vi "Parameter.vi"(9 "In":string, 10 "VIId":string, 11 "VariablesRef":T1) -> ()   [LabVIEW 2018, in "Time.lvlib"]
uses:
  Time.lvlib
  <userlib>/_OpenG.lib/dictionary/dictionary.llb/Dictionary Object RefNum__ogtk.ctl
  <userlib>/_OpenG.lib/dictionary/dictionary.llb/Dictionary Object RefNum - Enum__ogtk.ctl
  <vilib>/addons/_JKI.lib/Serialization/JSON/JKI JSON Serialization.lvlib
panel:
  in  "Tab Control":enum32{"Config", "控件"}(tab)
  in  "ArrayType":enum32{"Wait_ms", "Wait_s", "TickCount"}(tab)
  in  "时间(ms)":i32
  in  "时间(s)":i32
  in  "方法(Method)":enum16{"Wait_ms", "Wait_s", "TickCount"}(ring)
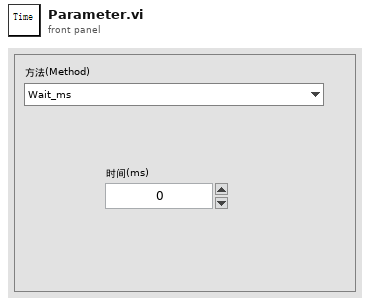
[diagram p1: front panel]
types:
  T1 = typedef "Dictionary Object RefNum__ogtk.ctl" = refnum<k1>
  T2 = cluster{"Wait_ms":cluster{"json":cluster{"Method":string, "Time":i32}}, "Wait_s":cluster{"json":cluster{"Method":string, "Time":i32}}, "TickCount":cluster{"json":cluster{"Method":string}}}
  T3 = enum32{"Invalid", "Standard", "Closed", "Hidden", "Minimized", "Maximized"}
  T4 = enum32{"invalid app kind", "Development System", "Run Time System", "Student Edition", "Embedded LabVIEW", "Evaluation", "Custom"}
  T5 = cluster{"Core":cluster{"Current VI Reference":refnum<vi>, "Close Panel on Exit?":bool}, "Parameter":cluster{"VariableRef":T1}, "Synchronize":cluster{"EnqueueData":cluster{"Action":enum16{"Create", "Query", "Revert", "UpdateVariable", "Close"}, "Data":variant}, "Echo":cluster{"VIRef":refnum<vi>, "JsonOut":string, "Status":string}, "Communicate":cluster{"ID":string, "JsonIn":string, "VarRef":T1}, "Queue":refnum<queue>}, "TimeClusters":cluster{"Wait_ms":cluster{"json":cluster{"Method":string, "Time":i32}}, "Wait_s":cluster{"json":cluster{"Method":string, "Time":i32}}, "TickCount":cluster{"json":cluster{"Method":string}}}}
  T6 = cluster{"EnqueueData":cluster{"Action":enum16{"Create", "Query", "Revert", "UpdateVariable", "Close"}, "Data":variant}, "Echo":cluster{"VIRef":refnum<vi>, "JsonOut":string, "Status":string}, "Communicate":cluster{"ID":string, "JsonIn":string, "VarRef":T1}, "Queue":refnum<queue>}
  T7 = cluster{"Current VI Reference":refnum<vi>, "Close Panel on Exit?":bool}
  T8 = cluster{"json":cluster{"Method":string, "Time":i32}}
  T9 = cluster{"Action":enum16{"Create", "Query", "Revert", "UpdateVariable", "Close"}, "Data":variant}
  T10 = cluster{"ID":string, "JsonIn":string, "VarRef":T1}
  T11 = enum16{"Create", "Query", "Revert", "UpdateVariable", "Close"}
  T12 = cluster{"VIRef":refnum<vi>, "JsonOut":string, "Status":string}
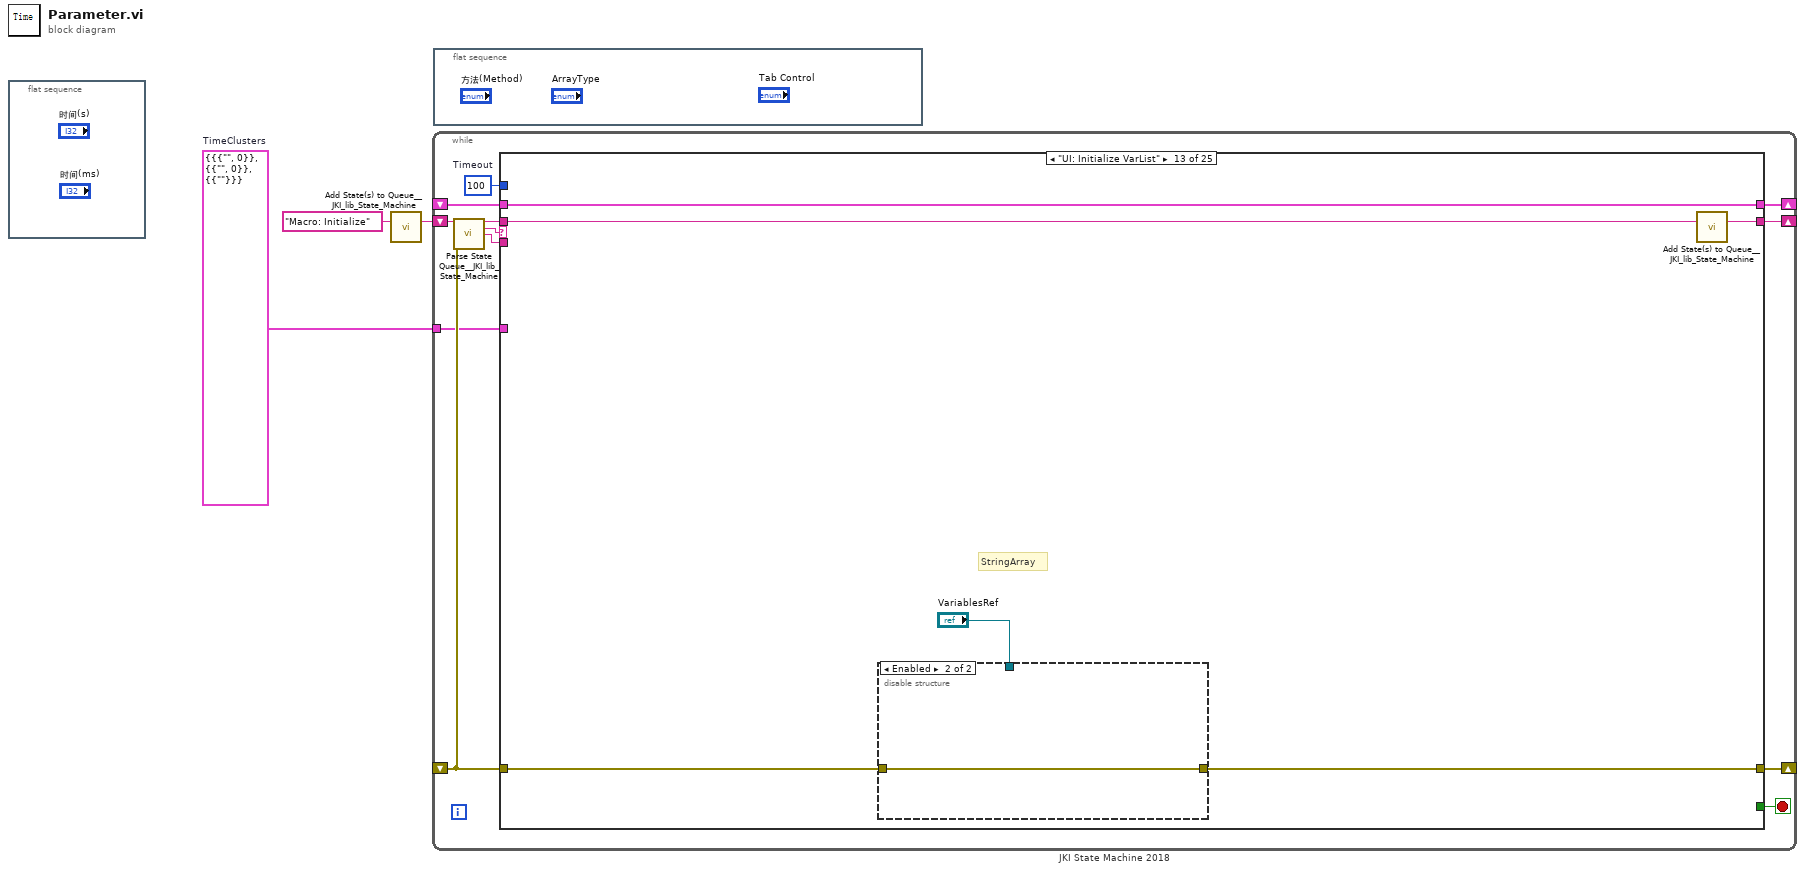
[diagram p0: block diagram]
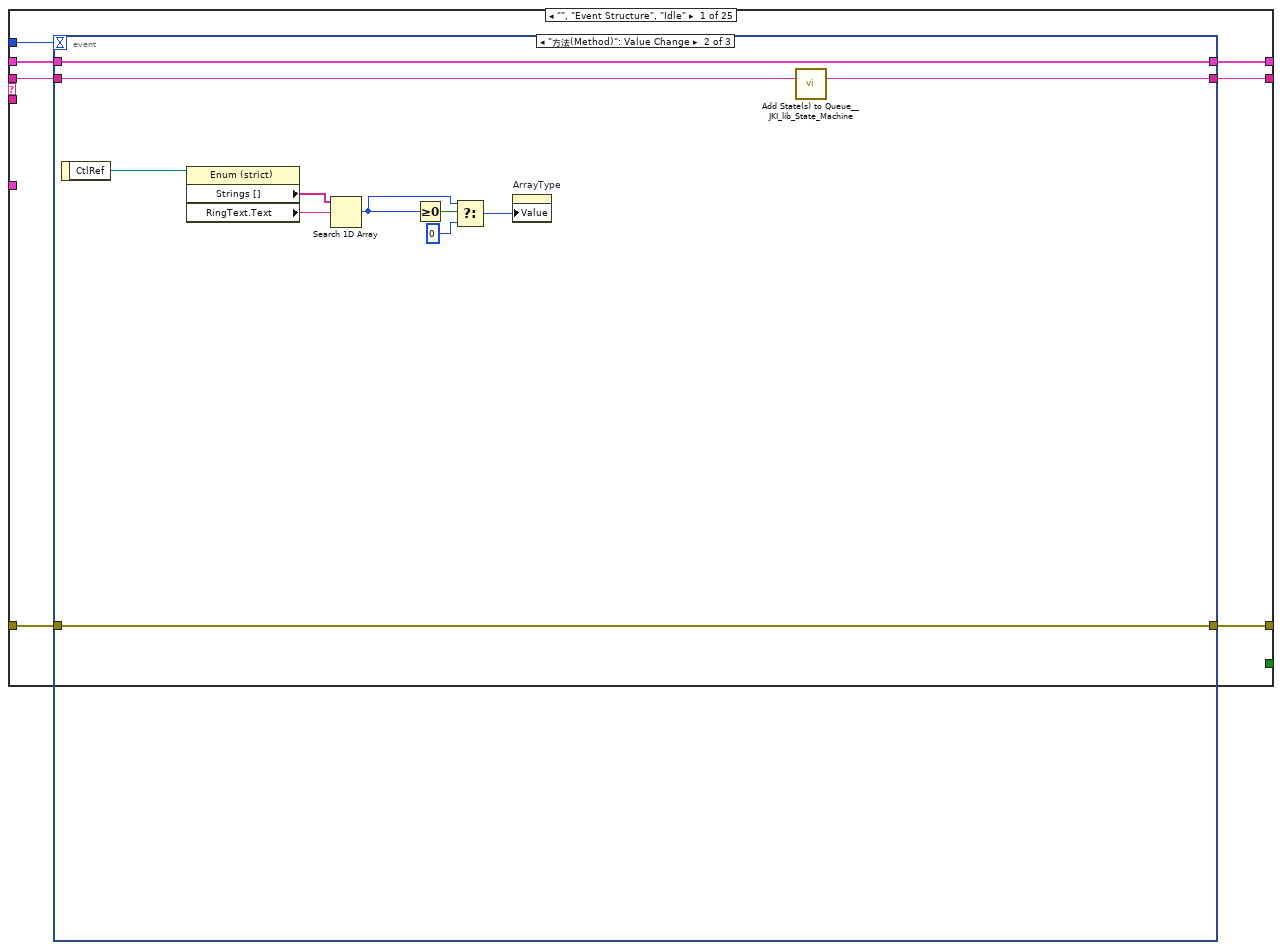
[diagram p2: hidden frame]
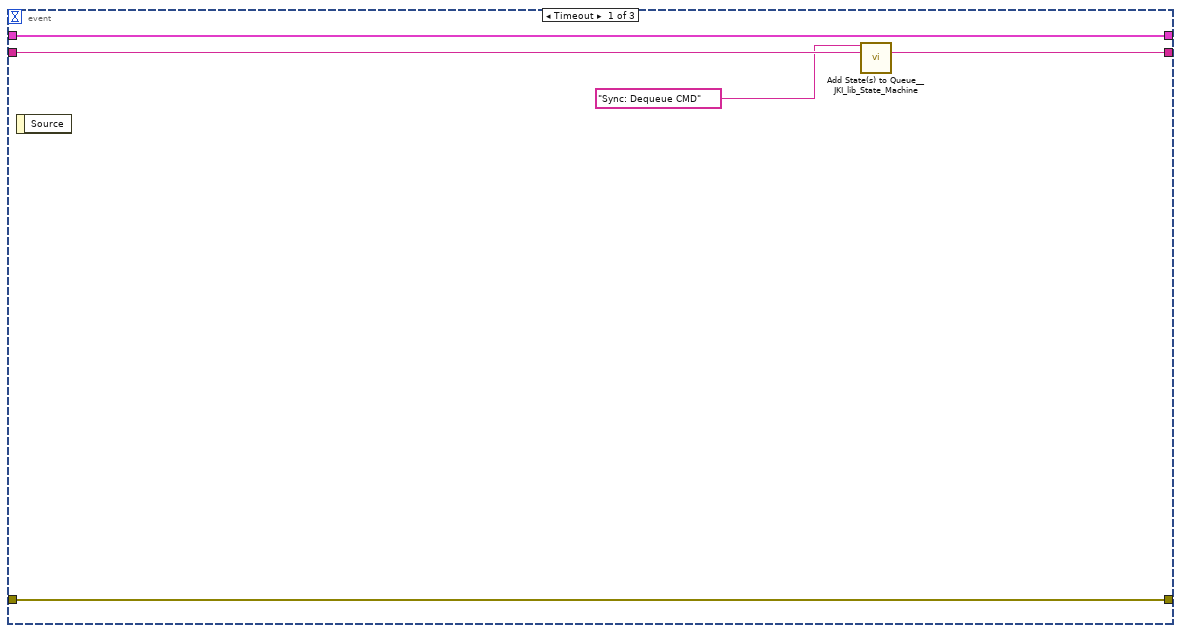
[diagram p3: hidden frame]
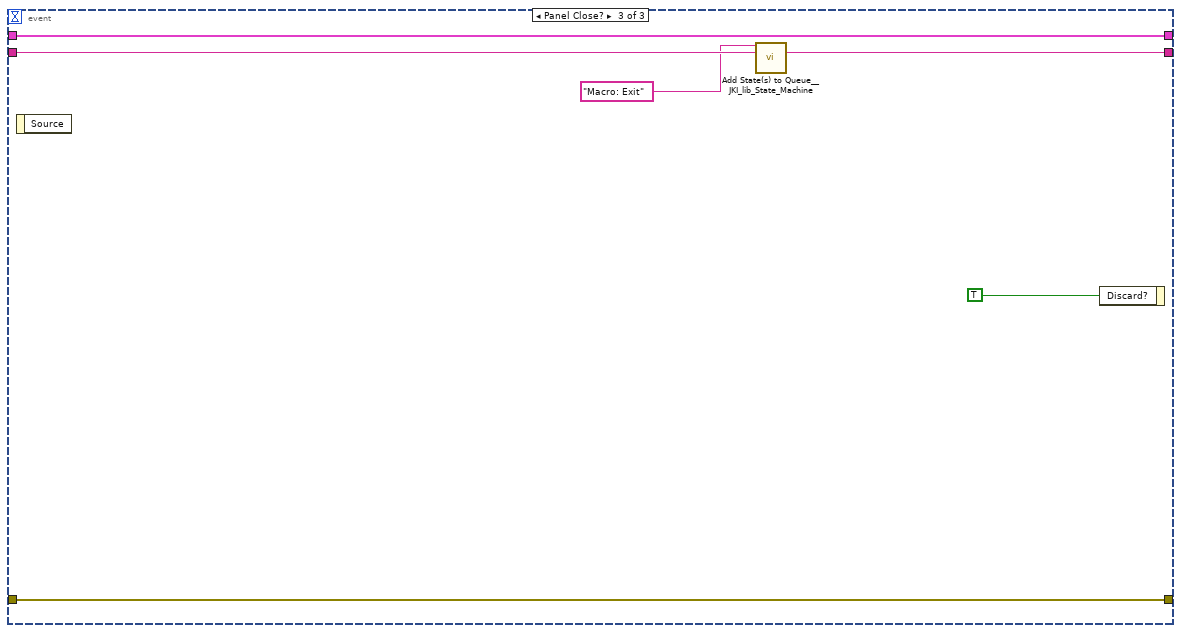
[diagram p4: hidden frame]
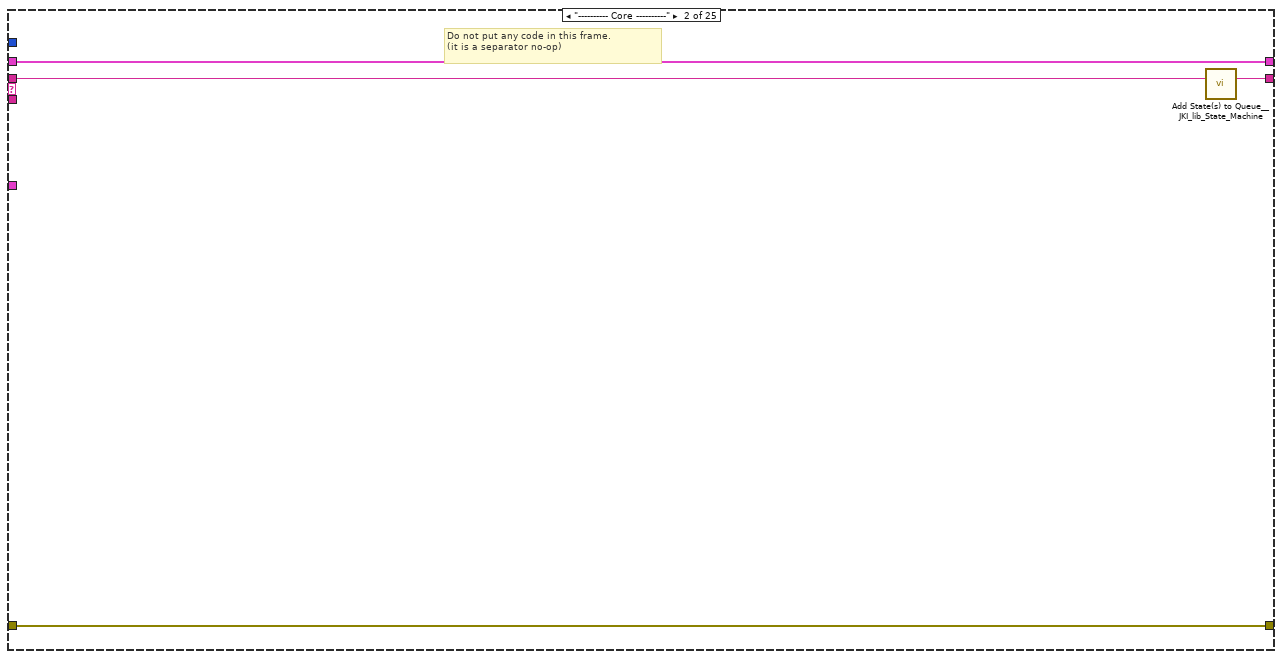
[diagram p5: hidden frame]
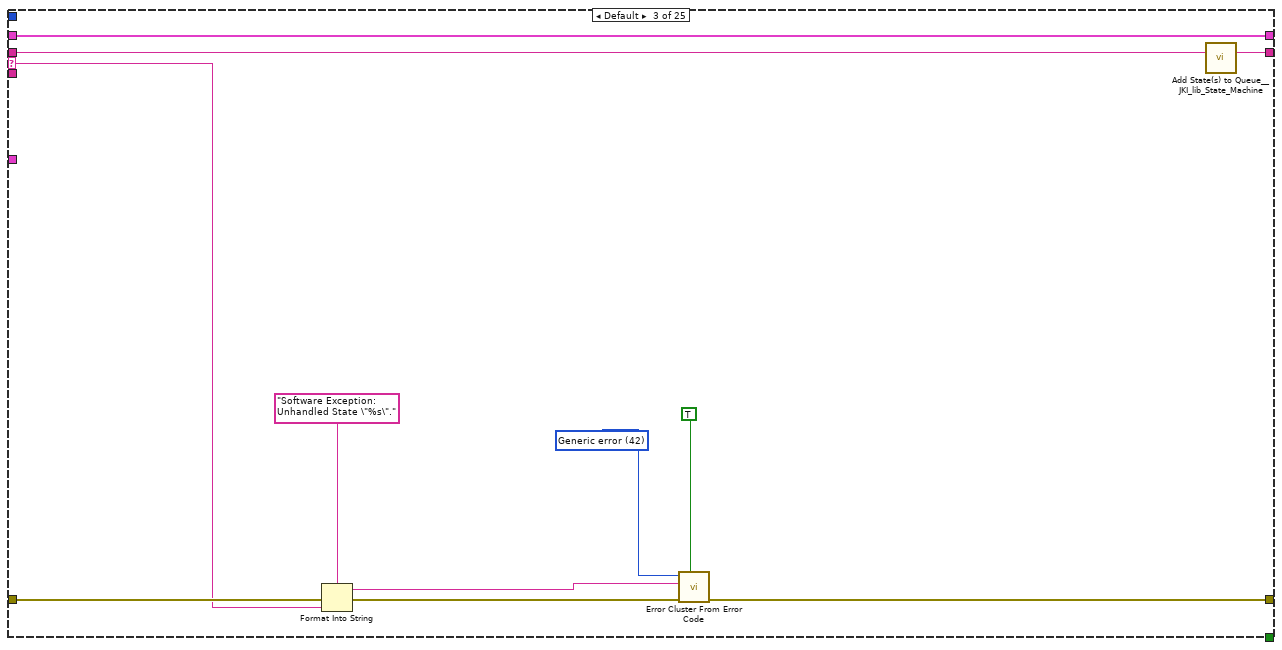
[diagram p6: hidden frame]
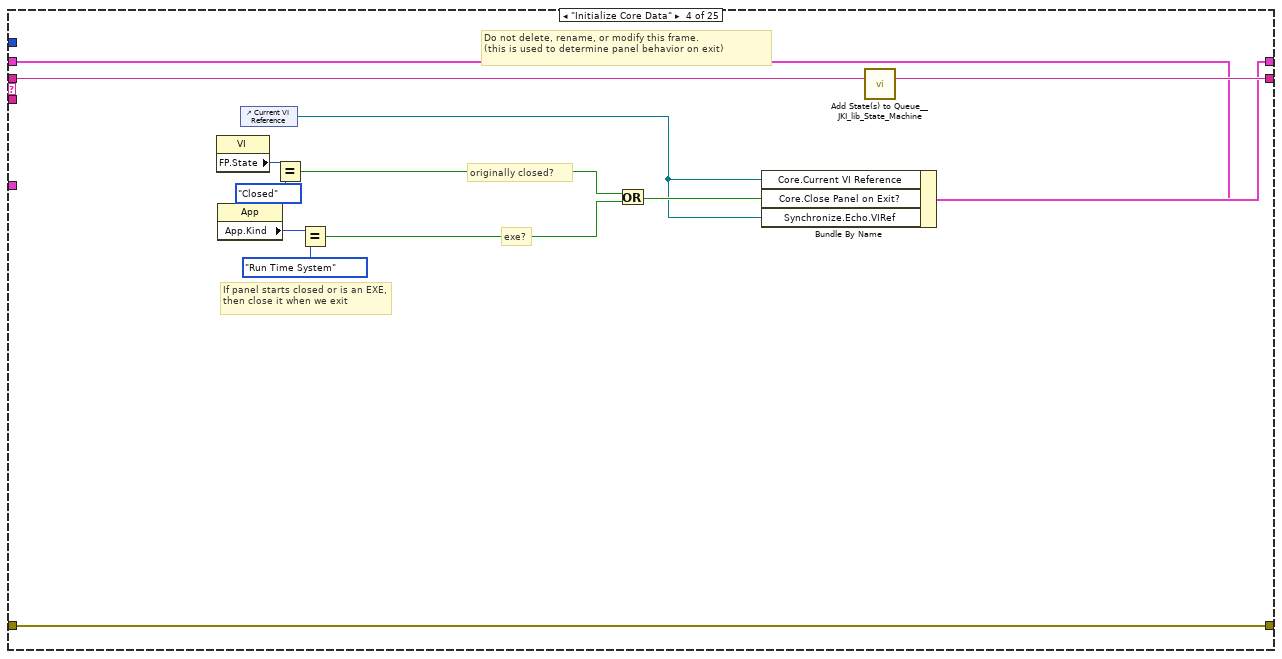
[diagram p7: hidden frame]
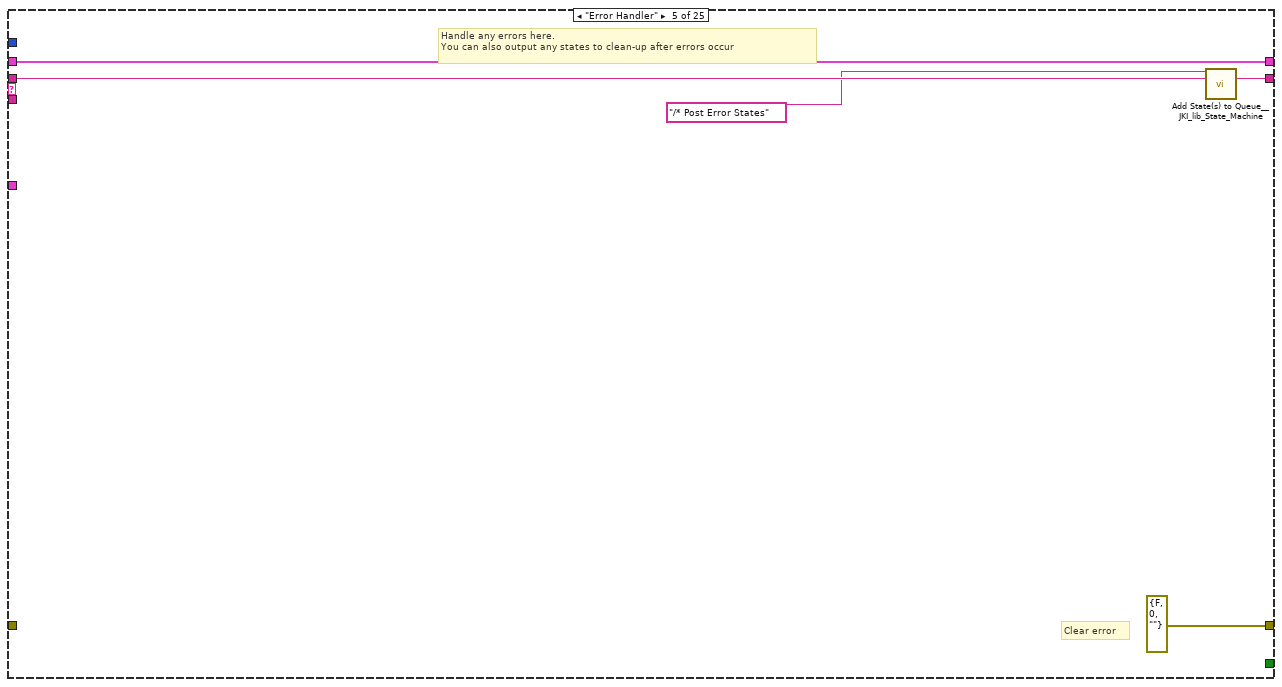
[diagram p8: hidden frame]
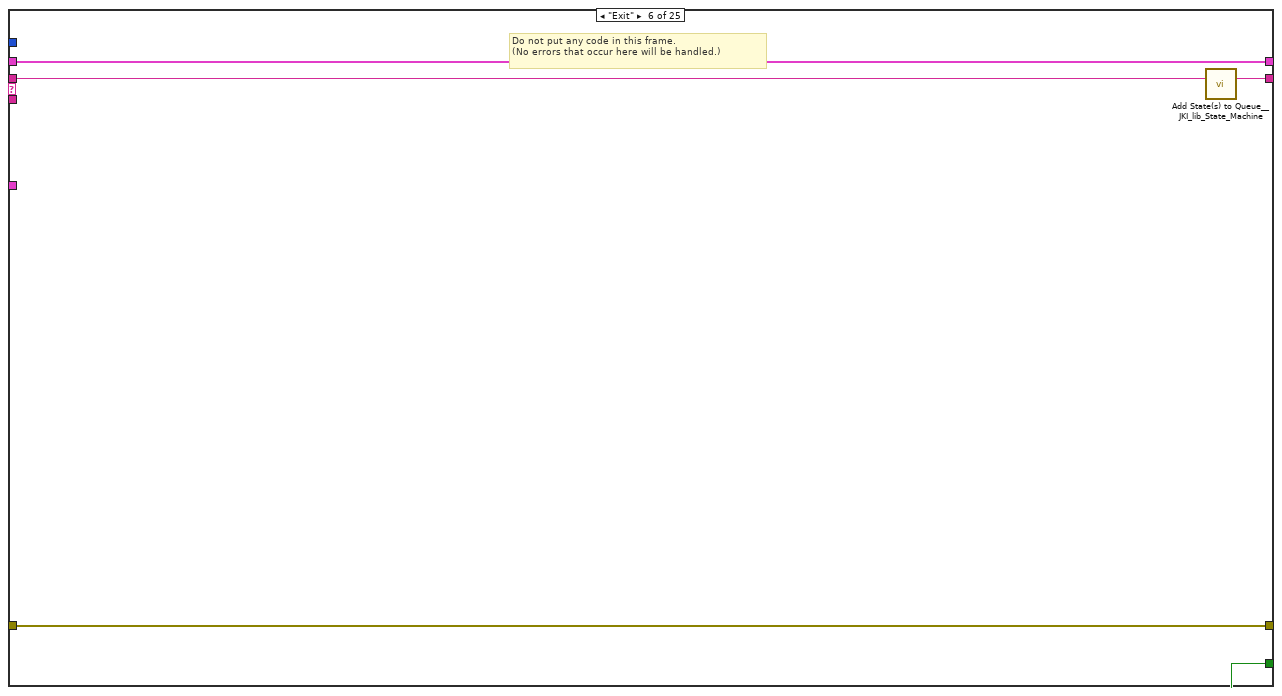
[diagram p9: hidden frame]
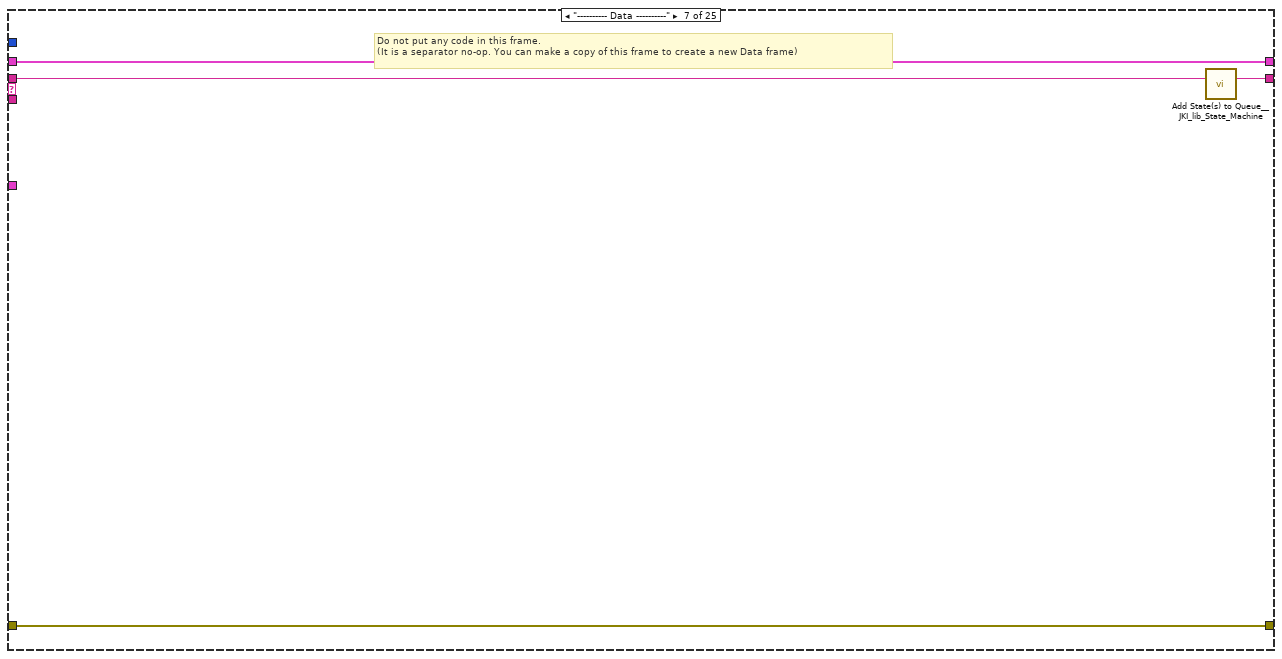
[diagram p10: hidden frame]
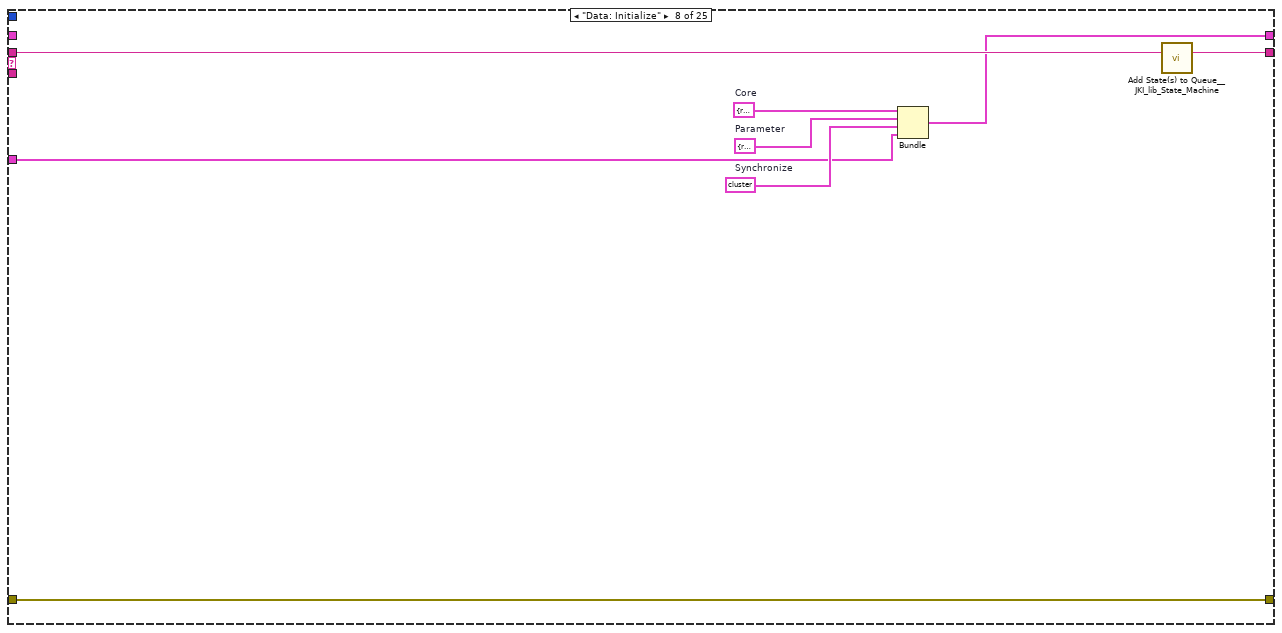
[diagram p11: hidden frame]
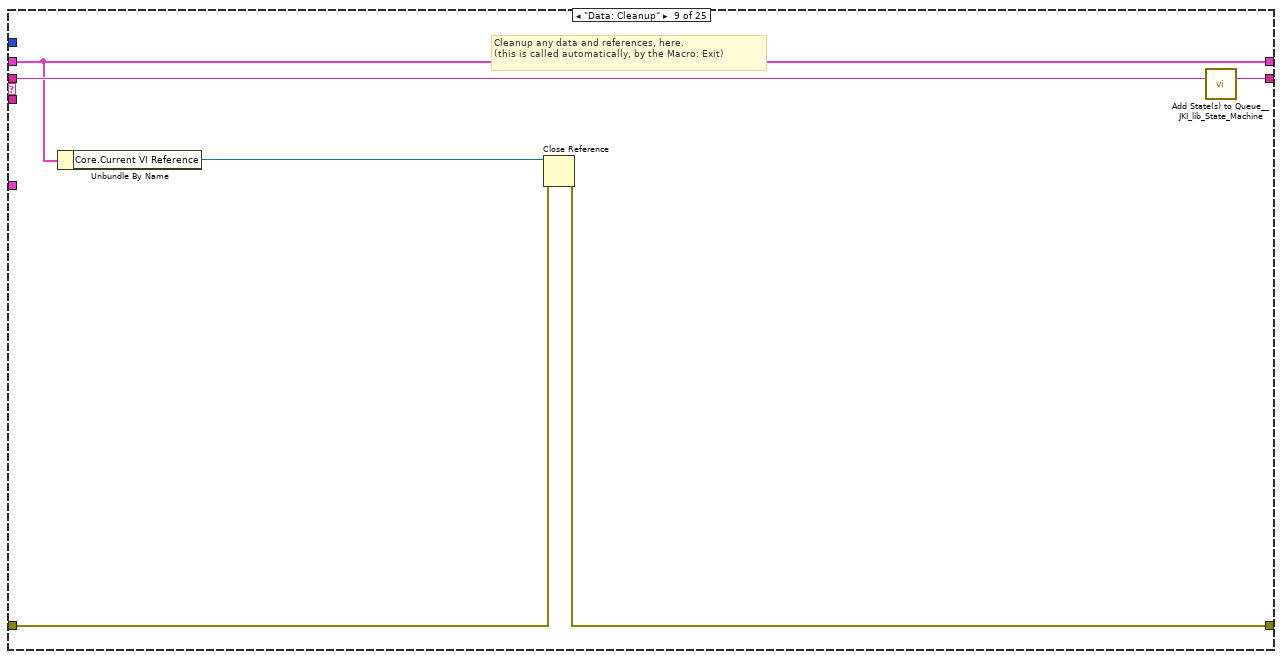
[diagram p12: hidden frame]
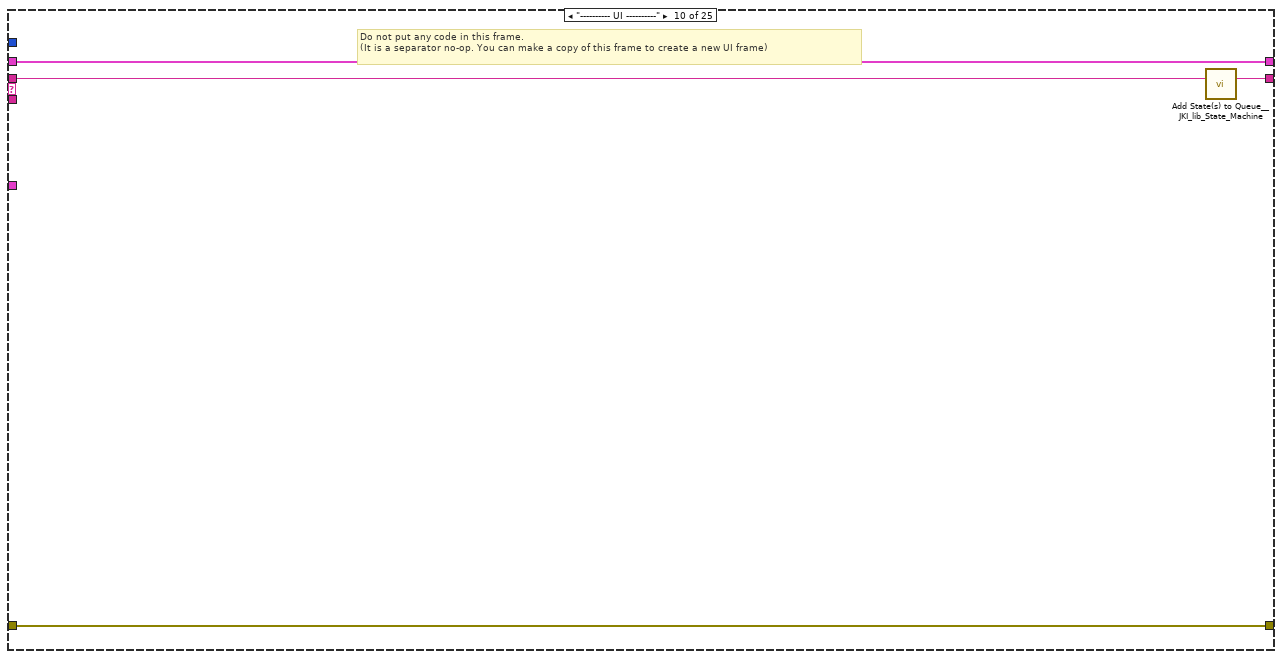
[diagram p13: hidden frame]
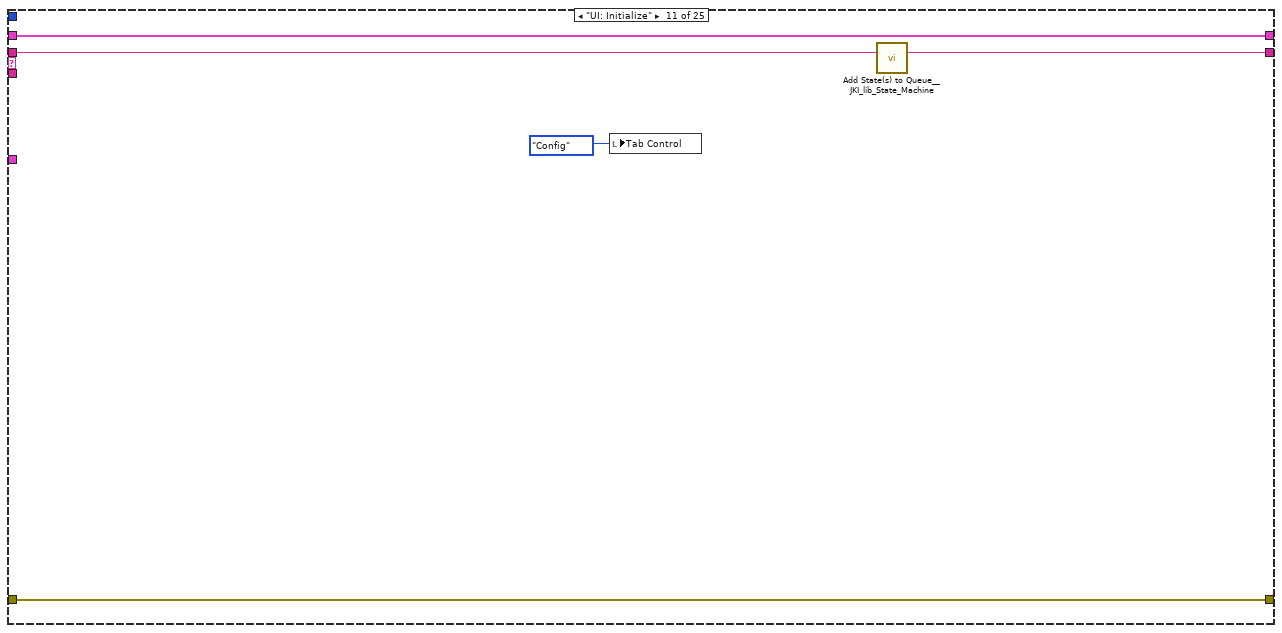
[diagram p14: hidden frame]
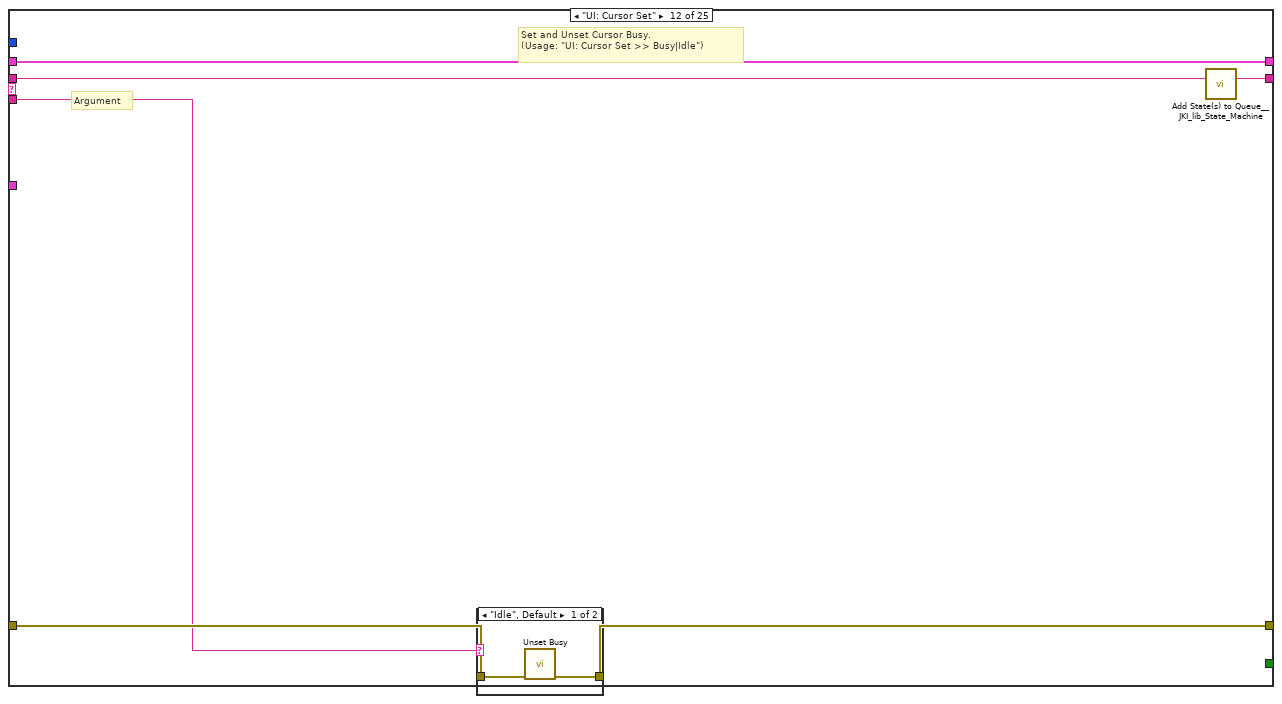
[diagram p15: hidden frame]
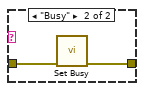
[diagram p16: hidden frame]
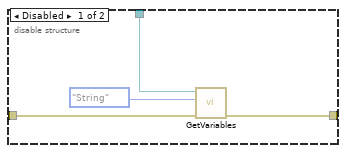
[diagram p17: hidden frame]
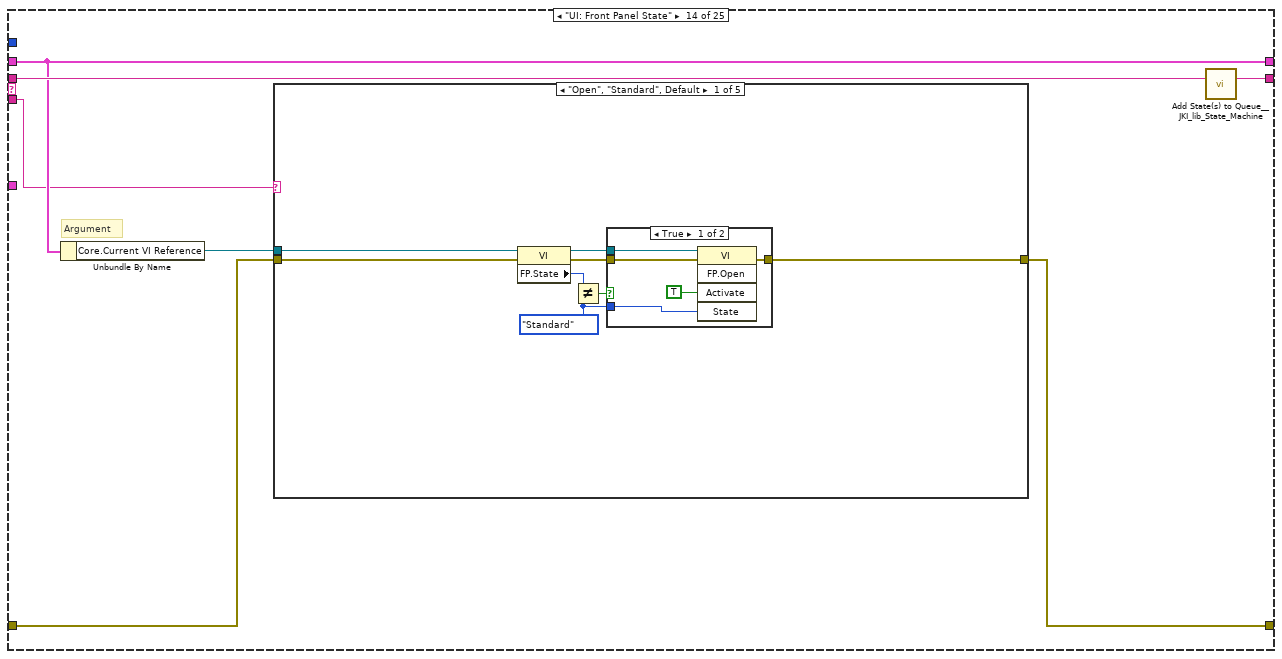
[diagram p18: hidden frame]
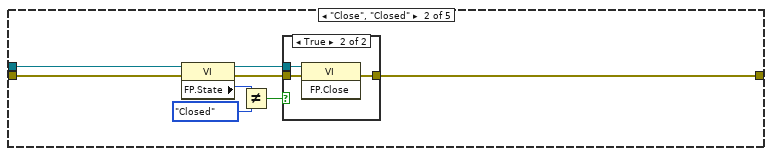
[diagram p20: hidden frame]
diagram:
  w1 = T2 {"Wait_ms"={"json"={"Method"="", "Time"=0}}, "Wait_s"={"json"={"Method"="", "Time"=0}}, "TickCount"={"json"={"Method"=""}}}  # TimeClusters
  n1 = flat-sequence {
    frame #0 {
    }
  }
  n2 = call <vilib>:"Add State(s) to Queue__JKI_lib_State_Machine.vi"("State(s) in (\"\")"="Macro: Initialize") -> ("States Out"=w3:string)  [unwired: 14 in]
  n3 = while "JKI State Machine 2018" {
    shift-right: [w8] -> _
    shift-left: _ -> [w7]
    shift-right: [w11] -> _
    shift-left: _ -> [w5]
    shift-right: [w10] -> _
    shift-left: w3 -> [w12]
    tunnel: w1 -> [w4]
    stop <- w9 stop-if-true
    w6 = 100  # Timeout
    n4 = call <vilib>:"Parse State Queue__JKI_lib_State_Machine.vi"("State Queue"=w12, "Error In (no error)"=w5) -> ("Remaining States"=w14:string, "Current State"=w15:string, "Arguments"=w13:string)  [unwired: 11 in]
    n5 = case shown="\"UI: Initialize VarList\"" w15 {
      selector: w15 -> [_ _ w49 _ _ _ _ _ _ _ _ _ _ _ _ _ _ _ _ _ _ _ _ _ _]
      tunnel: w14 -> [w22 w48 w53 w72 w77 w82 w86 w94 w100 w104 w109 w115 w125 w137 w206 w211 w221 w225 w233 w287 w318 w327 w342 w386 w401]
      tunnel: w13 -> [_ _ _ _ _ _ _ _ _ _ _ w110 _ w131 _ _ _ _ _ _ _ _ _ _ _]
      tunnel: w7 -> [w20 w45 w51 w65 w74 w80 w83 _ w95 w101 w106 w113 w123 w133 w203 w208 w218 w222 w228 w280 w315 w320 w340 w383 w390]
      tunnel: [w19 w46 w55 w69 errorcluster {"status"=FALSE, "code"=0, "source"=""} ("error out") w79 w84 w92 w96 w102 w105 w111 w120 w134 w204 w209 w219 w223 w229 w284 w316 w324 w329 w381 w388] -> w11
      tunnel: w5 -> [w18 w46 w54 w69 _ w79 w84 w92 w97 w102 w105 w112 w121 w135 w204 w209 w219 w223 w230 w283 w316 w325 w338 w382 w389]
      tunnel: [w21 w47 w52 w71 w76 w81 w85 w93 w99 w103 w108 w114 w124 w136 w205 w210 w220 w224 w232 w286 w317 w326 w341 w385 w400] -> w10
      tunnel: [_ _ _ _ _ TRUE _ _ _ _ _ _ _ _ _ _ _ _ _ _ _ _ _ _ _] -> w9
      tunnel: [w17 w45 w51 w70 w74 w80 w83 w89 w95 w101 w106 w113 w123 w133 w203 w208 w218 w222 w228 w285 w315 w322 w331 w383 w390] -> w8
      tunnel: w6 -> [w16 _ _ _ _ _ _ _ _ _ _ _ _ _ _ _ _ _ _ _ _ _ _ _ _]
      tunnel: w4 -> [_ _ _ _ _ _ _ w87 _ _ _ _ _ _ _ _ _ _ _ _ _ _ _ _ _]
      frame "", "Event Structure", "Idle" {
        n6 = event shown="[1] \"方法(Method)\": Value Change" {
          selector: _ -> [_ _ _]
          dyn-events: _ -> [_ _ _]
          timeout: w16 -> [_ _ _]
          tunnel: w22 -> [w27 w38 w44]
          tunnel: [w26 w37 w43] -> w21
          tunnel: w20 -> [w24 w35 w41]
          tunnel: [w25 w36 w42] -> w19
          tunnel: w18 -> [w25 w36 w42]
          tunnel: [w24 w35 w41] -> w17
          event Timeout {
            n7 = event-data() -> ()  [unwired: 1 in, 1 out]
            n8 = call <vilib>:"Add State(s) to Queue__JKI_lib_State_Machine.vi"("State(s) in Front (\"\")"="Sync: Dequeue CMD" ("State(s) in Front (\"\")"), "State(s) in (\"\")"=w27) -> ("States Out"=w26:string)  [unwired: 13 in]
          }
          event "方法(Method)": Value Change {
            n9 = event-data() -> ("CtlRef"=w31:refnum<vi>)  [unwired: 1 in]
            n10 = property class="Enum (strict)"(reference=w31) -> ("Strings []"=w30:string[], "RingText.Text"=w29:string)  [unwired: 1 in, 2 out]
            n11 = Search 1D Array(1D array=w30, element=w29) -> (index of element=w33:i32)  [unwired: 1 in]
            n12 = Greater Or Equal To 0?(x=w33) -> (x >= 0?=w34:bool)
            n13 = Select(t=w33, s=w34, f=0) -> (s? t:f=w28:i32)
            n14 = property on="ArrayType" class="TabCtl (strict)"("Value"=w28) -> ()  [unwired: 2 in, 2 out]
            n15 = call <vilib>:"Add State(s) to Queue__JKI_lib_State_Machine.vi"("State(s) in (\"\")"=w38) -> ("States Out"=w37:string)  [unwired: 14 in]
          }
          event Panel Close? {
            n16 = event-data() -> ()  [unwired: 1 in, 1 out]
            n17 = call <vilib>:"Add State(s) to Queue__JKI_lib_State_Machine.vi"("State(s) in Front (\"\")"="Macro: Exit", "State(s) in (\"\")"=w44) -> ("States Out"=w43:string)  [unwired: 13 in]
            n18 = event-data("Discard?"=TRUE) -> ()  [unwired: 1 in, 1 out]
          }
        }
      }
      frame "---------- Core ----------" {
        # "Do not put any code in this frame.\n(it is a separator no-op)"
        n19 = call <vilib>:"Add State(s) to Queue__JKI_lib_State_Machine.vi"("State(s) in (\"\")"=w48) -> ("States Out"=w47:string)  [unwired: 14 in]
      }
      frame Default {
        w58 = 42 items=["No error", "Argument error", "Memory is full", "Out of zone", "End of file", "File already open", "Generic file I/O error", "File not found", "File permission error", "Disk is full", "Duplicate path", "Too many files open", "System feature not enabled", "Resource file not found", "Cannot add resource", "Resource not found", "Image not found", "Image memory error", "Pen does not exist", "Config type invalid", "Config token not found", "Config parse error", "Config memory error", "Bad external code format", "Bad external code offset", "External code not present", "Null window", "Destroy window error", "Null menu", "Print aborted", "Bad print record", "Print driver error", "Windows error during printing", "Memory error during printing", "Print dialog error", "Generic print error", "Invalid device refnum", "Device not found", "Device parameter error", "Device unit error", "Cannot open device", "Device call aborted", "Generic error", "Cancelled by user", "Object ID too low", "Object ID too high", "Object not in heap", "Unknown heap", "Unknown object (invalid DefProc)", "Unknown object (DefProc not in table)", "Message out of range", "Invalid (null) method", "Unknown message", "Manager call not supported", "Bad address", "Network operation in progress", "Network operation timed out", "Connection is busy", "Network attribute not supported", "Network error", "Address in use", "System out of memory", "Connection aborted", "Connection refused", "Not connected", "Already connected", "Connection closed", "Initialization error (interapplication manager)", "Bad occurrence", "Wait on unbound occurrence handler", "Occurrence queue overflow", "Datalog type conflict", "Unused", "Unrecognized type (interapplication manager)", "Memory corrupt", "Failed to make temporary DLL", "Old CIN version", "Drag socket not found", "Failed to load drop-object", "Failed to register OLE object", "Failed to release OLE object", "Format specifier type mismatch", "Unknown format specifier", "Too few format specifiers", "Too many format specifiers", "Scan failed", "Newer CIN version", "Error converting to variant", "Runtime menu error", "Password tampered", "Variant attribute not found", "Incompatible variant data type", "Event data is not available", "Event Store is not present", "Occurrence is not found", "Event Queue is not created", "Event info is not available", "Refnum passed is NULL", "Error retrieving Class GUID", "Error retrieving CoClass GUID", "Error retrieving TypeLib GUID.", "Bad built application magic bytes.", "Specific driver is different from the specific driver associated with the Logical Name.", "There is no session opened to the class driver.", "Max Error", "MAX - Error with config objects", "MAX - Error loading configuration", "MAX - Group not supported"]
        n20 = Format Into String(format string="Software Exception: Unhandled State \"%s\"." ("message"), error in=w54, w49) -> (resulting string=w57:string, error out=w56:errorcluster)  [unwired: 1 in]
        n21 = call <vilib>:"Error Cluster From Error Code.vi"("show call chain? (False)"=TRUE, "error in (no error)"=w56, "error message (\"\")"=w57, "error code (0)"=w58) -> ("error out"=w55:errorcluster)  [unwired: 5 in]
        n22 = call <vilib>:"Add State(s) to Queue__JKI_lib_State_Machine.vi"("State(s) in (\"\")"=w53) -> ("States Out"=w52:string)  [unwired: 14 in]
      }
      frame "Initialize Core Data" {
        # "Do not delete, rename, or modify this frame.\n(this is used to determine panel behavior on exit)"
        # "originally closed?"
        # "exe?"
        # "If panel starts closed or is an EXE, then close it when we exit"
        n23 = property class="VI"() -> ("FP.State"=w63:T3)  [unwired: 2 in, 2 out]
        n24 = property class="App"() -> ("App.Kind"=w68:T4)  [unwired: 2 in, 2 out]
        n25 = control-ref of="Current VI Reference"() -> (w60:refnum<vi>)
        n26 = Equal?(x=w63, y=T3."Closed" ("Front Panel Window:State")) -> (x = y?=w61:bool)
        n27 = Equal?(x=w68, y=T4."Run Time System" ("Application:Kind")) -> (x = y?=w66:bool)
        n28 = Or(x=w61, y=w66) -> (x .or. y?=w64:bool)
        n29 = Bundle By Name(cluster=w65, "Core.Current VI Reference"=w60, "Core.Close Panel on Exit?"=w64, "Synchronize.Echo.VIRef"=w60) -> (w70:T5)
        n30 = call <vilib>:"Add State(s) to Queue__JKI_lib_State_Machine.vi"("State(s) in (\"\")"=w72) -> ("States Out"=w71:string)  [unwired: 14 in]
      }
      frame "Error Handler" {
        # "Handle any errors here.\nYou can also output any states to clean-up after errors occur"
        # "Clear error"
        n31 = call <vilib>:"Add State(s) to Queue__JKI_lib_State_Machine.vi"("State(s) in Front (\"\")"="/* Post Error States", "State(s) in (\"\")"=w77) -> ("States Out"=w76:string)  [unwired: 13 in]
      }
      frame "Exit" {
        # "Do not put any code in this frame.\n(No errors that occur here will be handled.)"
        n32 = call <vilib>:"Add State(s) to Queue__JKI_lib_State_Machine.vi"("State(s) in (\"\")"=w82) -> ("States Out"=w81:string)  [unwired: 14 in]
      }
      frame "---------- Data ----------" {
        # "Do not put any code in this frame.\n(It is a separator no-op. You can make a copy of this frame to create a new Data frame)"
        n33 = call <vilib>:"Add State(s) to Queue__JKI_lib_State_Machine.vi"("State(s) in (\"\")"=w86) -> ("States Out"=w85:string)  [unwired: 14 in]
      }
      frame "Data: Initialize" {
        w88 = cluster{"VariableRef":T1} {"VariableRef"=refnum}  # Parameter
        w90 = T6 {"EnqueueData"={"Action"=enum."Create", "Data"=variant}, "Echo"={"VIRef"=refnum, "JsonOut"="", "Status"=""}, "Communicate"={"ID"="", "JsonIn"="", "VarRef"=refnum}, "Queue"=refnum}  # Synchronize
        w91 = T7 {"Current VI Reference"=refnum, "Close Panel on Exit?"=FALSE}  # Core
        n34 = Bundle("Core"=w91, "Parameter"=w88, "Synchronize"=w90, "TimeClusters"=w87) -> (w89:T5)  [unwired: 1 in]
        n35 = call <vilib>:"Add State(s) to Queue__JKI_lib_State_Machine.vi"("State(s) in (\"\")"=w94) -> ("States Out"=w93:string)  [unwired: 14 in]
      }
      frame "Data: Cleanup" {
        # "Cleanup any data and references, here.\n(this is called automatically, by the Macro: Exit)"
        n36 = Unbundle By Name(w95) -> ("Core.Current VI Reference"=w98:refnum<vi>)
        n37 = Close Reference(reference=w98, error in (no error)=w97) -> (error out=w96:errorcluster)
        n38 = call <vilib>:"Add State(s) to Queue__JKI_lib_State_Machine.vi"("State(s) in (\"\")"=w100) -> ("States Out"=w99:string)  [unwired: 14 in]
      }
      frame "---------- UI ----------" {
        # "Do not put any code in this frame.\n(It is a separator no-op. You can make a copy of this frame to create a new UI frame)"
        n39 = call <vilib>:"Add State(s) to Queue__JKI_lib_State_Machine.vi"("State(s) in (\"\")"=w104) -> ("States Out"=w103:string)  [unwired: 14 in]
      }
      frame "UI: Initialize" {
        n40 = local write "Tab Control"(enum32{"Config", "控件"}."Config" ("Tab Control")) -> ()
        n41 = call <vilib>:"Add State(s) to Queue__JKI_lib_State_Machine.vi"("State(s) in (\"\")"=w109) -> ("States Out"=w108:string)  [unwired: 14 in]
      }
      frame "UI: Cursor Set" {
        # "Argument"
        # "Set and Unset Cursor Busy.\n(Usage: \"UI: Cursor Set >> Busy|Idle\")"
        n42 = case shown="\"Idle\", Default" w110 {
          tunnel: w112 -> [w117 w119]
          tunnel: [w116 w118] -> w111
          frame "Idle", Default {
            n43 = call <vilib>:"Unset Busy.vi"("error in (no error)"=w117) -> ("error out"=w116:errorcluster)  [unwired: 10 in]
          }
          frame "Busy" {
            n44 = call <vilib>:"Set Busy.vi"("error in (no error)"=w119) -> ("error out"=w118:errorcluster)  [unwired: 9 in, 1 out]
          }
        }
        n45 = call <vilib>:"Add State(s) to Queue__JKI_lib_State_Machine.vi"("State(s) in (\"\")"=w115) -> ("States Out"=w114:string)  [unwired: 14 in]
      }
      frame "UI: Initialize VarList" {
        # "StringArray"
        n46 = disable-structure shown="Enabled" {
          disable-tunnel: "VariablesRef" -> [w129 _]
          disable-tunnel: w121 -> [w127 w130]
          disable-tunnel: [w126 w130] -> w120
          frame Disabled {
            n47 = call "GetVariables.vi"("error in (no error)"=w127, "VariableType"=enum16{"String", "StringArray"}."String", "DicRef"=w129) -> ("error out"=w126:errorcluster)  [unwired: 7 in, 1 out]
          }
          frame Enabled {
          }
        }
        n48 = call <vilib>:"Add State(s) to Queue__JKI_lib_State_Machine.vi"("State(s) in (\"\")"=w125) -> ("States Out"=w124:string)  [unwired: 14 in]
      }
      frame "UI: Front Panel State" {
        # "Argument"
        n49 = Unbundle By Name(w133) -> ("Core.Current VI Reference"=w132:refnum<vi>)
        n50 = case shown="\"Open\", \"Standard\", Default" w131 {
          tunnel: w135 -> [w143 w158 w169 w182 w195]
          tunnel: [w145 w159 w171 w184 w197] -> w134
          tunnel: w132 -> [w144 w156 w170 w183 w196]
          frame "Open", "Standard", Default {
            w138 = T3."Standard" ("State")
            n51 = property class="VI"(reference=w144, error in=w143) -> (reference out=w141:refnum<vi>, error out=w142:errorcluster, "FP.State"=w140:T3)
            n52 = Not Equal?(x=w140, y=w138) -> (x != y?=w139:bool)
            n53 = case shown="True" w139 {
              tunnel: [w149 w151] -> w145
              tunnel: w142 -> [w148 w151]
              tunnel: w141 -> [w147 _]
              tunnel: w138 -> [w146 _]
              frame True {
                n54 = invoke class="VI" method="FP.Open"(reference=w147, error in=w148, "Activate"=TRUE, "State"=w146) -> (error out=w149:errorcluster)  [unwired: 1 in, 4 out]
              }
              frame False {
              }
            }
          }
          frame "Close", "Closed" {
            n55 = property class="VI"(reference=w156, error in=w158) -> (reference out=w155:refnum<vi>, error out=w157:errorcluster, "FP.State"=w153:T3)
            n56 = Not Equal?(x=w153, y=T3."Closed" ("Front Panel Window:State")) -> (x != y?=w152:bool)
            n57 = case shown="True" w152 {
              tunnel: [w160 w163] -> w159
              tunnel: w157 -> [w160 w162]
              tunnel: w155 -> [_ w161]
              frame False {
              }
              frame True {
                n58 = invoke class="VI" method="FP.Close"(reference=w161, error in=w162) -> (error out=w163:errorcluster)  [unwired: 1 in, 2 out]
              }
            }
          }
          frame "Hidden", "Hide" {
            w164 = T3."Hidden" ("State")
            n59 = property class="VI"(reference=w170, error in=w169) -> (reference out=w167:refnum<vi>, error out=w168:errorcluster, "FP.State"=w166:T3)
            n60 = Not Equal?(x=w166, y=w164) -> (x != y?=w165:bool)
            n61 = case shown="True" w165 {
              tunnel: [w175 w176] -> w171
              tunnel: w168 -> [w174 w176]
              tunnel: w167 -> [w173 _]
              tunnel: w164 -> [w172 _]
              frame True {
                n62 = invoke class="VI" method="FP.Open"(reference=w173, error in=w174, "State"=w172) -> (error out=w175:errorcluster)  [unwired: 2 in, 4 out]
              }
              frame False {
              }
            }
          }
          frame "Minimize", "Minimized" {
            w177 = T3."Minimized" ("State")
            n63 = property class="VI"(reference=w183, error in=w182) -> (reference out=w180:refnum<vi>, error out=w181:errorcluster, "FP.State"=w179:T3)
            n64 = Not Equal?(x=w179, y=w177) -> (x != y?=w178:bool)
            n65 = case shown="True" w178 {
              tunnel: [w188 w189] -> w184
              tunnel: w181 -> [w187 w189]
              tunnel: w180 -> [w186 _]
              tunnel: w177 -> [w185 _]
              frame True {
                n66 = invoke class="VI" method="FP.Open"(reference=w186, error in=w187, "State"=w185) -> (error out=w188:errorcluster)  [unwired: 2 in, 4 out]
              }
              frame False {
              }
            }
          }
          frame "Maximize", "Maximized" {
            w190 = T3."Maximized" ("State")
            n67 = property class="VI"(reference=w196, error in=w195) -> (reference out=w193:refnum<vi>, error out=w194:errorcluster, "FP.State"=w192:T3)
            n68 = Not Equal?(x=w192, y=w190) -> (x != y?=w191:bool)
            n69 = case shown="True" w191 {
              tunnel: [w201 w202] -> w197
              tunnel: w194 -> [w200 w202]
              tunnel: w193 -> [w199 _]
              tunnel: w190 -> [w198 _]
              frame True {
                n70 = invoke class="VI" method="FP.Open"(reference=w199, error in=w200, "State"=w198) -> (error out=w201:errorcluster)  [unwired: 2 in, 4 out]
              }
              frame False {
              }
            }
          }
        }
        n71 = call <vilib>:"Add State(s) to Queue__JKI_lib_State_Machine.vi"("State(s) in (\"\")"=w137) -> ("States Out"=w136:string)  [unwired: 14 in]
      }
      frame "---------- Macro ----------" {
        n72 = call <vilib>:"Add State(s) to Queue__JKI_lib_State_Machine.vi"("State(s) in (\"\")"=w206) -> ("States Out"=w205:string)  [unwired: 14 in]
      }
      frame "Macro: Initialize" {
        n73 = call <vilib>:"Add State(s) to Queue__JKI_lib_State_Machine.vi"("State(s) in Front (\"\")"="Data: Initialize\nInitialize Core Data\nUI: Initialize\nSync: Obtain CMD Queue\nSync: Dequeue CMD\nUI: Initialize VarList\nParameter: Parse Parameter", "State(s) in (\"\")"=w211) -> ("States Out"=w210:string)  [unwired: 13 in]
      }
      frame "Macro: Exit" {
        n74 = Unbundle By Name(w218) -> ("Core.Close Panel on Exit?"=w217:bool)
        n75 = Select(t="UI: Front Panel State >> Close", s=w217, f="") -> (s? t:f=w214:string)
        n76 = call <vilib>:"Add State(s) to Queue__JKI_lib_State_Machine.vi"("State(s) in (\"\")"=w214, "State(s) at Back (\"\")"="Sync: Release CMD Queue\nData: Cleanup\nExit") -> ("States Out"=w212:string)  [unwired: 13 in]
        n77 = call <vilib>:"Add State(s) to Queue__JKI_lib_State_Machine.vi"("State(s) in Front (\"\")"=w212, "State(s) in (\"\")"=w221) -> ("States Out"=w220:string)  [unwired: 13 in]
      }
      frame "---------- Parameter ----------" {
        # "Template Separator\n(You can make a copy of, or modify, this frame)"
        n78 = call <vilib>:"Add State(s) to Queue__JKI_lib_State_Machine.vi"("State(s) in (\"\")"=w225) -> ("States Out"=w224:string)  [unwired: 14 in]
      }
      frame "Parameter: Parse Parameter" {
        n79 = Unbundle By Name(w228) -> ("TimeClusters"=w227:T2)
        n80 = Empty String/Path?(string/path="In") -> (empty?=w231:bool)
        n81 = case shown="False" w231 {
          tunnel: "In" -> [w242 _]
          tunnel: w230 -> [w247 w278]
          tunnel: [w246 w278] -> w229
          tunnel: w227 -> [w245 _]
          frame False {
            n82 = Match Pattern(string=w242, regular expression="\"Method\":\"") -> (after substring=w241:string)  [unwired: 1 in, 3 out]
            n83 = Match Pattern(string=w241, regular expression="\",") -> (before substring=w240:string)  [unwired: 1 in, 3 out]
            n84 = case shown="\"TickCount\"" w240 {
              tunnel: w242 -> [w255 w265 w274 _]
              tunnel: w247 -> [w253 w263 w272 w277]
              tunnel: [w252 w262 w271 w277] -> w246
              tunnel: w245 -> [w250 w260 w269 _]
              tunnel: [w251 w261 w270 _] -> w235
              frame "Wait_ms" {
                n85 = Unbundle By Name(w250) -> ("Wait_ms"=w249:T8)
                n86 = call <vilib>:"Unflatten From JSON String.vi"("Type and Defaults"=w249, "error in (no error)"=w253, "JSON String"=w255) -> ("error out"=w256:errorcluster, "Variant"=w257:variant)  [unwired: 7 in]
                n87 = Variant To Data(error in=w256, type=w249, Variant=w257) -> (data=w254:T8, error out=w252:errorcluster)
                n88 = Unbundle By Name(w254) -> ("json.Method"=w251:string, "json.Time"=w248:i32)
                n89 = local write "时间(ms)"(w248) -> ()
              }
              frame "Wait_s" {
                n90 = Unbundle By Name(w260) -> ("Wait_s"=w259:T8)
                n91 = call <vilib>:"Unflatten From JSON String.vi"("Type and Defaults"=w259, "error in (no error)"=w263, "JSON String"=w265) -> ("error out"=w266:errorcluster, "Variant"=w267:variant)  [unwired: 7 in]
                n92 = Variant To Data(error in=w266, type=w259, Variant=w267) -> (data=w264:T8, error out=w262:errorcluster)
                n93 = Unbundle By Name(w264) -> ("json.Method"=w261:string, "json.Time"=w258:i32)
                n94 = local write "时间(ms)"(w258) -> ()
              }
              frame "TickCount" {
                n95 = Unbundle By Name(w269) -> ("TickCount"=w268:cluster{"json":cluster{"Method":string}})
                n96 = call <vilib>:"Unflatten From JSON String.vi"("Type and Defaults"=w268, "error in (no error)"=w272, "JSON String"=w274) -> ("error out"=w275:errorcluster, "Variant"=w276:variant)  [unwired: 7 in]
                n97 = Variant To Data(error in=w275, type=w268, Variant=w276) -> (data=w273:cluster{"json":cluster{"Method":string}}, error out=w271:errorcluster)
                n98 = Unbundle By Name(w273) -> ("json.Method"=w270:string)
              }
              frame Default {
              }
            }
            n99 = property on="方法(Method)" class="Enum (strict)"() -> ("Strings []"=w237:string[])  [unwired: 2 in, 2 out]
            n100 = Search 1D Array(1D array=w237, element=w235) -> (index of element=w239:i32)  [unwired: 1 in]
            n101 = Greater Or Equal To 0?(x=w239) -> (x >= 0?=w238:bool)
            n102 = Select(t=w239, s=w238, f=0) -> (s? t:f=w234:i32)
            n103 = local write "ArrayType"(w234) -> ()
            n104 = property on="方法(Method)" class="Enum (strict)"("Value"=w234) -> ()  [unwired: 2 in, 2 out]
          }
          frame True {
          }
        }
        n105 = call <vilib>:"Add State(s) to Queue__JKI_lib_State_Machine.vi"("State(s) in (\"\")"=w233) -> ("States Out"=w232:string)  [unwired: 14 in]
      }
      frame "Parameter: Combin Parameter" {
        n106 = property on="方法(Method)" class="Enum (strict)"() -> ("RingText.Text"=w282:string)  [unwired: 2 in, 2 out]
        n107 = Unbundle By Name(w280) -> ("TimeClusters"=w279:T2)
        n108 = case shown="\"TickCount\"" w282 {
          selector: w282 -> [_ w291 w300 w308]
          tunnel: w279 -> [_ w297 w306 w314]
          tunnel: [_ w295 w304 w312] -> w281
          tunnel: [w288 w290 w299 w307] -> w284
          tunnel: w283 -> [w288 w293 w302 w310]
          frame Default {
          }
          frame "Wait_ms" {
            n109 = Unbundle By Name(w297) -> ("Wait_ms"=w296:T8)
            n110 = local read "时间(ms)"() -> (w289:i32)
            n111 = Bundle By Name(cluster=w296, "json.Method"=w291, "json.Time"=w289) -> (w292:T8)
            n112 = call <vilib>:"Flatten To JSON String.vi"("Multiline (T)"=TRUE, "error in (no error)"=w293, "Variant"=w292) -> ("error out"=w290:errorcluster, "JSON String"=w295:string)  [unwired: 7 in]
          }
          frame "Wait_s" {
            n113 = Unbundle By Name(w306) -> ("Wait_s"=w305:T8)
            n114 = local read "时间(s)"() -> (w298:i32)
            n115 = Bundle By Name(cluster=w305, "json.Method"=w300, "json.Time"=w298) -> (w301:T8)
            n116 = call <vilib>:"Flatten To JSON String.vi"("Multiline (T)"=TRUE, "error in (no error)"=w302, "Variant"=w301) -> ("error out"=w299:errorcluster, "JSON String"=w304:string)  [unwired: 7 in]
          }
          frame "TickCount" {
            n117 = Unbundle By Name(w314) -> ("TickCount"=w313:cluster{"json":cluster{"Method":string}})
            n118 = Bundle By Name(cluster=w313, "json.Method"=w308) -> (w309:cluster{"json":cluster{"Method":string}})
            n119 = call <vilib>:"Flatten To JSON String.vi"("Multiline (T)"=TRUE, "error in (no error)"=w310, "Variant"=w309) -> ("error out"=w307:errorcluster, "JSON String"=w312:string)  [unwired: 7 in]
          }
        }
        n120 = Bundle By Name(cluster=w280, "Synchronize.Echo.JsonOut"=w281) -> (w285:T5)
        n121 = call <vilib>:"Add State(s) to Queue__JKI_lib_State_Machine.vi"("State(s) in (\"\")"=w287) -> ("States Out"=w286:string)  [unwired: 14 in]
      }
      frame "---------- Sync ----------" {
        n122 = call <vilib>:"Add State(s) to Queue__JKI_lib_State_Machine.vi"("State(s) in (\"\")"=w318) -> ("States Out"=w317:string)  [unwired: 14 in]
      }
      frame "Sync: Obtain CMD Queue" {
        # "这里由平台输入"
        n123 = Unbundle By Name(w320) -> ("Synchronize.EnqueueData"=w319:T9)
        n124 = Obtain Queue(name (unnamed)="VIId", element data type=w319, error in (no error)=w325) -> (queue out=w321:refnum<queue>, error out=w324:errorcluster)  [unwired: 2 in, 1 out]
        n125 = Bundle By Name(cluster=w320, "Synchronize.Queue"=w321) -> (w322:T5)
        n126 = call <vilib>:"Add State(s) to Queue__JKI_lib_State_Machine.vi"("State(s) in (\"\")"=w327) -> ("States Out"=w326:string)  [unwired: 14 in]
      }
      frame "Sync: Dequeue CMD" {
        n127 = Unbundle By Name(w340) -> ("Synchronize.Queue"=w337:refnum<queue>, "Synchronize.Communicate"=w328:T10)
        n128 = Dequeue Element(queue=w337, timeout in ms (-1)=10, error in (no error)=w338) -> (queue out=w336:refnum<queue>, element=w334:T9, timed out?=w335:bool, error out=w330:errorcluster)
        n129 = Bundle By Name(cluster=w340, "Synchronize.Queue"=w336, "Synchronize.EnqueueData"=w334) -> (w332:T5)
        n130 = case shown="False" w335 {
          tunnel: w334 -> [w351 _]
          tunnel: [w349 _] -> w333
          tunnel: w332 -> [w348 w380]
          tunnel: [w347 w380] -> w331
          tunnel: w330 -> [w345 w379]
          tunnel: [w344 w379] -> w329
          tunnel: w328 -> [w343 _]
          frame False {
            n131 = Unbundle By Name(w351) -> ("Action"=w350:T11, "Data"=w346:variant)
            n132 = case shown="\"Query\"" w350 {
              tunnel: ["Sync: Send ECHO" "UI: Initialize VarList\nSync: Send ECHO" _ "Sync: Send ECHO\nMacro: Exit" "Parameter: Combin Parameter\nSync: Send ECHO" "Parameter: Parse Parameter\nSync: Send ECHO"] -> w349
              tunnel: w348 -> [w354 w359 w363 w366 w371 w376]
              tunnel: [w353 w358 w363 w365 w370 w375] -> w347
              tunnel: w346 -> [_ _ _ _ _ _]
              tunnel: w345 -> [w355 w360 w362 w367 w372 w377]
              tunnel: [w355 w360 w362 w367 w372 w377] -> w344
              tunnel: w343 -> [_ _ _ _ _ _]
              frame "Create" {
                n133 = Bundle By Name(cluster=w354, "Synchronize.Echo.Status"="Create Success") -> (w353:T5)
              }
              frame "UpdateVariable" {
                n134 = Bundle By Name(cluster=w359, "Synchronize.Echo.Status"="UpdateVariable Success") -> (w358:T5)
              }
              frame Default {
              }
              frame "Close" {
                n135 = Bundle By Name(cluster=w366, "Synchronize.Echo.Status"="Close Success") -> (w365:T5)
              }
              frame "Query" {
                n136 = Bundle By Name(cluster=w371, "Synchronize.Echo.Status"="Query Success") -> (w370:T5)
              }
              frame "Revert" {
                n137 = Bundle By Name(cluster=w376, "Synchronize.Echo.Status"="Revert Success") -> (w375:T5)
              }
            }
          }
          frame True {
          }
        }
        n138 = call <vilib>:"Add State(s) to Queue__JKI_lib_State_Machine.vi"("State(s) in Front (\"\")"=w333, "State(s) in (\"\")"=w342) -> ("States Out"=w341:string)  [unwired: 13 in]
      }
      frame "Sync: Release CMD Queue" {
        n139 = Unbundle By Name(w383) -> ("Synchronize.Queue"=w384:refnum<queue>)
        n140 = Release Queue(queue=w384, error in (no error)=w382) -> (error out=w381:errorcluster)  [unwired: 1 in, 2 out]
        n141 = call <vilib>:"Add State(s) to Queue__JKI_lib_State_Machine.vi"("State(s) in (\"\")"=w386) -> ("States Out"=w385:string)  [unwired: 14 in]
      }
      frame "Sync: Send ECHO" {
        n142 = Unbundle By Name(w390) -> ("Synchronize.Communicate"=w387:T10, "Synchronize.EnqueueData.Data"=w399:variant, "Synchronize.Echo"=w391:T12)
        n143 = Variant To Data(error in=w389, type=w387, Variant=w399) -> (data=w392:T10, error out=w393:errorcluster)
        n144 = Unbundle By Name(w392) -> ("ID"=w396:string)
        n145 = Obtain Queue(name (unnamed)=w396, element data type=w391, error in (no error)=w393) -> (queue out=w395:refnum<queue>, error out=w397:errorcluster)  [unwired: 2 in, 1 out]
        n146 = Enqueue Element(queue=w395, element=w391, error in (no error)=w397) -> (queue out=w394:refnum<queue>, error out=w398:errorcluster)  [unwired: 1 in, 1 out]
        n147 = Release Queue(queue=w394, error in (no error)=w398) -> (error out=w388:errorcluster)  [unwired: 1 in, 2 out]
        n148 = call <vilib>:"Add State(s) to Queue__JKI_lib_State_Machine.vi"("State(s) in (\"\")"=w401) -> ("States Out"=w400:string)  [unwired: 14 in]
      }
    }
  }
  n149 = flat-sequence {
    frame #0 {
    }
  }
